vi "WorkorderHandler_getDataToModify.vi"(0 "reference":T1, 3 "timeout in ms (-1)":i32=-1, 5 "error in (no error)":errorcluster) -> (14 "duplicate reference":T1, 16 "data":T2, 18 "timed out?":bool, 19 "error out":errorcluster)   [LabVIEW 2011]
doc: "Returns the data of dqGOOP object and locks it"
uses:
  DataStructures/WorkorderHandler_ObjectReference.ctl
  DataStructures/WorkorderHandler_ObjectData.ctl
panel:
  in  "queue (default)":refnum<queue>
  # "Copyright (C) 2004 DataAct Incorporated"
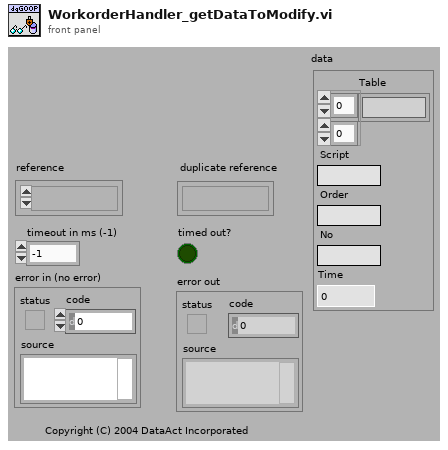
[diagram p1: front panel]
types:
  T1 = typedef "WorkorderHandler_ObjectReference.ctl" = refnum<k1>
  T2 = typedef "WorkorderHandler_ObjectData.ctl" = cluster{"Table":string[][], "Script":string, "Order":string, "No":string, "Time":dbl}
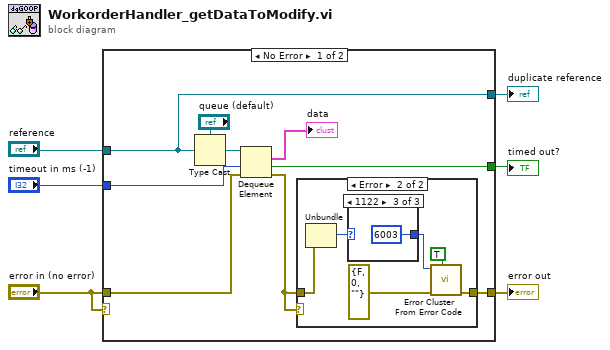
[diagram p0: block diagram]
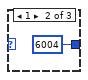
[diagram p4: hidden frame]
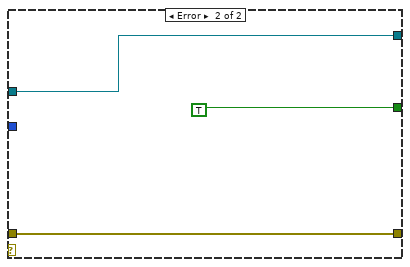
[diagram p5: hidden frame]
diagram:
  n1 = case shown="No Error" "error in (no error)" {
    tunnel: [w8 w26] -> w6
    tunnel: [w15 TRUE] -> w1
    tunnel: "reference" -> [w9 w27]
    tunnel: [w9 w27] -> w4
    tunnel: "timeout in ms (-1)" -> [w13 _]
    tunnel: "error in (no error)" -> [w12 w26]
    frame No Error {
      n2 = Type Cast(type="queue (default)", x=w9) -> (*(type *) &x=w10:refnum<queue>)
      n3 = Dequeue Element(queue=w10, timeout in ms (-1)=w13, error in (no error)=w12) -> (element=→"data":T2, timed out?=w15:bool, error out=w7:errorcluster)  [unwired: 1 out]
      n4 = case shown="Error" w7 {
        tunnel: [w16 w17] -> w8
        tunnel: w7 -> [w16 w22]
        frame No Error {
        }
        frame Error {
          n5 = Unbundle(w22) -> ("code"=w21:i32)  [unwired: 2 out]
          n6 = case shown="1122" w21 {
            selector: w21 -> [w23 _ _]
            tunnel: [w23 6004 ("code") 6003 ("code")] -> w19
            frame Default {
            }
            frame 1 {
            }
            frame 1122 {
            }
          }
          n7 = call <vilib>:"Error Cluster From Error Code.vi"("show call chain? (False)"=TRUE, "error in (no error)"=errorcluster {"status"=FALSE, "code"=0, "source"=""} ("error out"), "error code (0)"=w19) -> ("error out"=w17:errorcluster)  [unwired: 6 out]
        }
      }
    }
    frame Error {
    }
  }
  "error out" <- w6
  "duplicate reference" <- w4
  "timed out?" <- w1
